vi "FTW-Color-From HSL.vi"(1 "Luminance":dbl, 2 "Saturation":dbl, 3 "Hue":dbl) -> (0 "Color":u32(colorbox))   [LabVIEW 2015]
doc: "Converts a HSL (Hue, Saturation, Lumanence) color space color value into a 32 bit RGB (Red, Green, Blue) color space value."
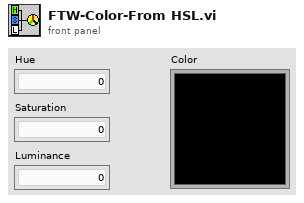
[diagram p1: front panel]
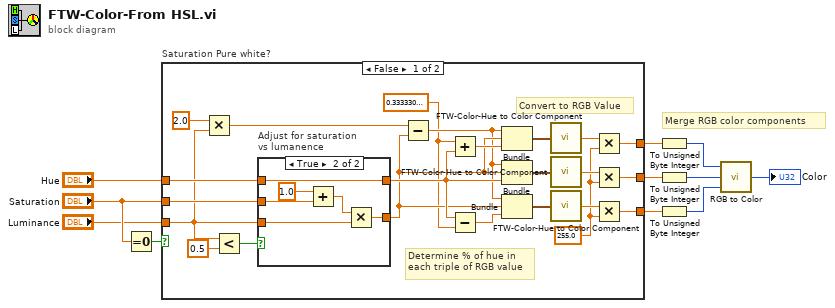
[diagram p0: block diagram]
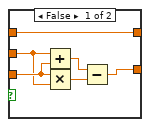
[diagram p2: hidden frame]
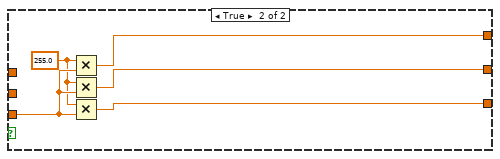
[diagram p3: hidden frame]
diagram:
  # "Merge RGB color components"
  n1 = Equal To 0?(x="Saturation") -> (x = 0?=w11:bool)
  n2 = case "Saturation Pure white?" shown="False" w11 {
    tunnel: "Luminance" -> [w30 w51]
    tunnel: "Saturation" -> [w33 _]
    tunnel: "Hue" -> [w32 _]
    tunnel: [w14 w47] -> w8
    tunnel: [w13 w48] -> w9
    tunnel: [w12 w49] -> w10
    frame False {
      w15 = 255.0 ("x")
      w22 = 0.3333300054073334 ("x")
      # "Convert to RGB Value"
      # "Determine % of hue in\neach triple of RGB value"
      n3 = Multiply(x=2.0, y=w30) -> (x*y=w28:dbl)
      n4 = Less?(x=w30, y=0.5) -> (x < y?=w31:bool)
      n5 = case "Adjust for saturation\nvs lumanence" shown="True" w31 {
        tunnel: w30 -> [w39 w42]
        tunnel: w33 -> [w38 w45]
        tunnel: w32 -> [w40 w46]
        tunnel: [w40 w46] -> w25
        tunnel: [w35 w41] -> w24
        frame False {
          n6 = Add(x=w38, y=w39) -> (x+y=w37:dbl)
          n7 = Multiply(x=w39, y=w38) -> (x*y=w36:dbl)
          n8 = Subtract(x=w37, y=w36) -> (x-y=w35:dbl)
        }
        frame True {
          n9 = Add(x=1.0, y=w45) -> (x+y=w43:dbl)
          n10 = Multiply(x=w43, y=w42) -> (x*y=w41:dbl)
        }
      }
      n11 = Subtract(x=w28, y=w24) -> (x-y=w23:dbl)
      n12 = Add(x=w22, y=w25) -> (x+y=w27:dbl)
      n13 = Subtract(x=w25, y=w22) -> (x-y=w26:dbl)
      n14 = Bundle(w23, w24, w27) -> (w21:cluster{dbl, dbl, dbl})  [unwired: 1 in]
      n15 = Bundle(w23, w24, "Hue"=w25) -> (w20:cluster{dbl, dbl, "Hue":dbl})  [unwired: 1 in]
      n16 = Bundle(w23, w24, w26) -> (w19:cluster{dbl, dbl, dbl})  [unwired: 1 in]
      n17 = call "FTW-Color-Hue to Color Component.vi"("Hue Vars"=w21) -> ("Color Component Value"=w18:dbl)
      n18 = call "FTW-Color-Hue to Color Component.vi"("Hue Vars"=w20) -> ("Color Component Value"=w17:dbl)
      n19 = call "FTW-Color-Hue to Color Component.vi"("Hue Vars"=w19) -> ("Color Component Value"=w16:dbl)
      n20 = Multiply(x=w18, y=w15) -> (x*y=w14:dbl)
      n21 = Multiply(x=w17, y=w15) -> (x*y=w13:dbl)
      n22 = Multiply(x=w16, y=w15) -> (x*y=w12:dbl)
    }
    frame True {
      w50 = sgl 255.0 ("x")
      n23 = Multiply(x=w50, y=w51) -> (x*y=w47:dbl)
      n24 = Multiply(x=w50, y=w51) -> (x*y=w48:dbl)
      n25 = Multiply(x=w50, y=w51) -> (x*y=w49:dbl)
    }
  }
  n26 = To Unsigned Byte Integer(number=w8) -> (unsigned 8bit integer=w6:u8)
  n27 = To Unsigned Byte Integer(number=w9) -> (unsigned 8bit integer=w7:u8)
  n28 = To Unsigned Byte Integer(number=w10) -> (unsigned 8bit integer=w5:u8)
  n29 = call <vilib>:"RGB to Color.vi"("B"=w5, "G"=w7, "R"=w6) -> ("Color"=→"Color":u32)
